vi "property_note.vi"() -> ()   [LabVIEW 2020]
panel:
  out "Number of Items":u32
  out "Ring Text.Text":string
  out "Strings []":string[](array[string])
  in  "SCIPI":u16(ring) items=["*IDN?", "*SAV 1 ", "*RCL 1 "]
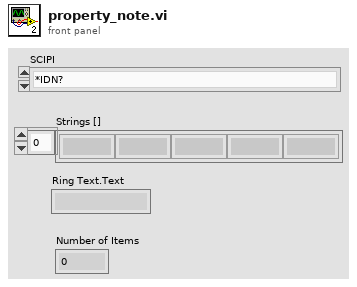
[diagram p1: front panel]
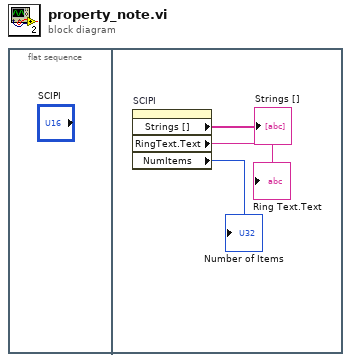
[diagram p0: block diagram]
diagram:
  n1 = flat-sequence {
    frame #0 {
    }
    frame #1 {
      n2 = property on="SCIPI" class="Ring (strict)"() -> ("Strings []"=→"Strings []":string[], "RingText.Text"=→"Ring Text.Text":string, "NumItems"=→"Number of Items":u32)  [unwired: 2 in, 2 out]
    }
  }
